vi "CounterTest_Program.vi"() -> ()   [LabVIEW 2014]
uses:
  Pixel Scan Parameters.ctl
panel:
  out "appended array":dbl[][](array[numeric])
  in  "Run":bool
  out "Normalized DM Pixel Value":dbl
  out "DM Pixel":u8
  in  "Pixel Scan Parameters In":T1={"Scan Start Pixel"=1, "Scan End Pixel"=1, "Pixel Start Value (-1 to 1)"=-0.5, "Pixel End Value (-1 to 1)"=0.5, "Number of Steps"=0.1}
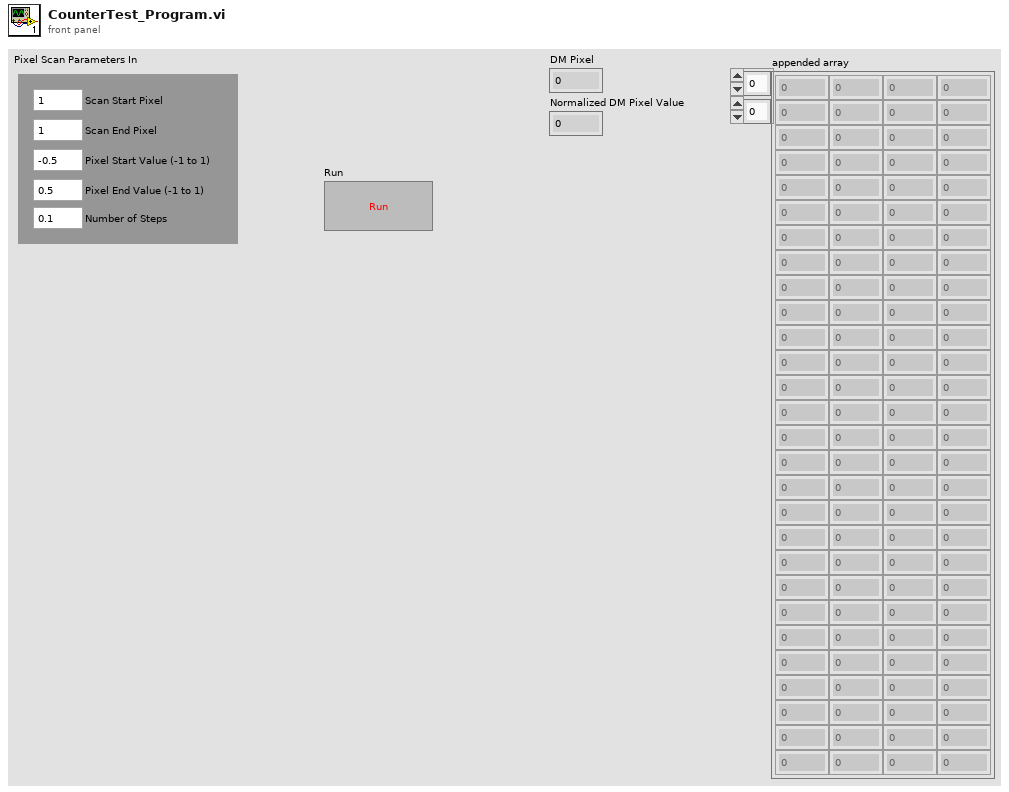
[diagram p1: front panel]
types:
  T1 = typedef "Pixel Scan Parameters.ctl" = cluster{"Scan Start Pixel":u8, "Scan End Pixel":u8, "Pixel Start Value (-1 to 1)":dbl, "Pixel End Value (-1 to 1)":dbl, "Number of Steps":dbl}
  T2 = enum16{"Reset Counter", "Update Counter", "Get Count"}
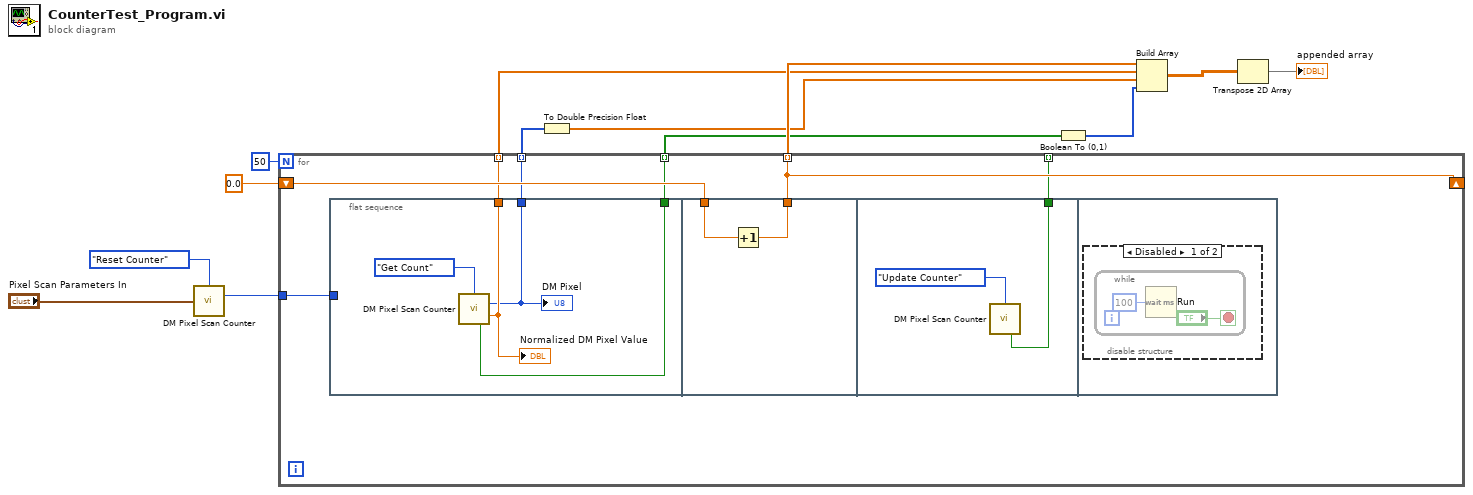
[diagram p0: block diagram]
diagram:
  n1 = call "DM Pixel Scan Counter.vi"("Action"=T2."Reset Counter", "Pixel Scan Parameters In"="Pixel Scan Parameters In") -> ("DM Pixel"=w11:u8)  [unwired: 11 in, 2 out]
  n2 = for {
    N: 50 -> [_]
    tunnel: w11 -> [w20]
    shift-right: [w17] -> _
    shift-left: 0.0 -> [w19]
    tunnel: [w17] -> w7 mode=indexing
    tunnel: [w18] -> w5 mode=indexing
    tunnel: [w16] -> w8 mode=indexing
    tunnel: [w15] -> _ mode=indexing
    tunnel: [w14] -> w1 mode=indexing
    n3 = flat-sequence {
      tunnel: w20 -> [_]
      tunnel: [w23] -> w18
      tunnel: [w22] -> w16
      tunnel: [w21] -> w14
      tunnel: w19 -> [w26]
      tunnel: [w25] -> w17
      tunnel: [w27] -> w15
      frame #0 {
        n4 = call "DM Pixel Scan Counter.vi"("Action"=T2."Get Count") -> ("DM Pixel"=w22:u8, "Normalized DM Pixel Value"=w23:dbl, "Scan Done"=w21:bool)  [unwired: 12 in]
        "DM Pixel" <- w22
        "Normalized DM Pixel Value" <- w23
      }
      frame #1 {
        n5 = Increment(x=w26) -> (x+1=w25:dbl)
      }
      frame #2 {
        n6 = call "DM Pixel Scan Counter.vi"("Action"=T2."Update Counter") -> ("Scan Done"=w27:bool)  [unwired: 12 in, 2 out]
      }
      frame #3 {
        n7 = disable-structure shown="Disabled" {
          frame Disabled {
            n8 = while {
              stop <- "Run" stop-if-true
              n9 = Wait (ms)(milliseconds to wait=u32 100) -> ()  [unwired: 1 out]
            }
          }
          frame Enabled {
          }
        }
      }
    }
  }
  n10 = To Double Precision Float(number=w8) -> (double precision float=w6:dbl[])
  n11 = Boolean To (0,1)(Boolean=w1) -> (0, 1=w2:i16[])
  n12 = Build Array(w7, w5, w6, w2) -> (w4:dbl[][])
  n13 = Transpose 2D Array(2D array=w4) -> (transposed array=→"appended array":dbl[][])
